vi "LED Color to bytes.vi"(11 "Array":u32[](array[colorbox])) -> ()   [LabVIEW 2026]
uses:
  MrcLib.lvlib
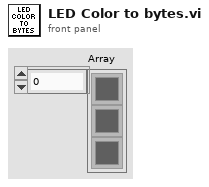
[diagram p1: front panel]
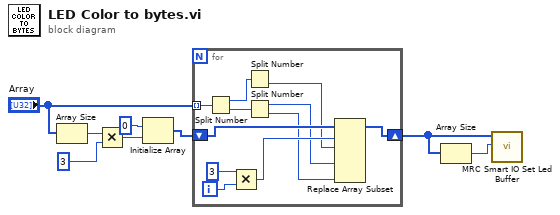
[diagram p0: block diagram]
diagram:
  n1 = Array Size(array="Array") -> (size(s)=w7:i32)
  n2 = Multiply(x=w7, y=3) -> (x*y=w5:i32)
  n3 = Initialize Array(u8 0 ("element"), w5) -> (w3:u8[])
  n4 = for {
    tunnel: "Array" -> [w17] mode=indexing
    shift-right: [w15] -> w1
    shift-left: w3 -> [w16]
    i -> [w14]
    n5 = Split Number(x=w17) -> (hi(x)=w19:u16, lo(x)=w18:u16)
    n6 = Multiply(x=3 ("y"), y=w14) -> (x*y=w12:i32)
    n7 = Split Number(x=w19) -> (lo(x)=w11:u8)  [unwired: 1 out]
    n8 = Split Number(x=w18) -> (hi(x)=w10:u8, lo(x)=w9:u8)
    n9 = Replace Array Subset(array=w16, new element #1=w11, index #1=w12, new element #2=w10, new element #3=w9) -> (w15:u8[])  [unwired: 2 in]
  }
  n10 = Array Size(array=w1) -> (size(s)=w2:i32)
  n11 = call "MRC Smart IO Set Led Buffer.vi"("bufferLength"=w2, "buffer Data"=w1) -> ()  [unwired: 9 in, 1 out]
